vi "LVDimInterface.dic_info_service.vi"   [LabVIEW 2014, in "LVDimInterface.lvlib"]
uses:
  LVDimInterface.lvlib
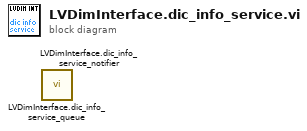
[diagram p0: block diagram]
diagram:
  n1 = call "LVDimInterface.dic_info_service_queue.vi"() -> ()  [unwired: 18 in, 2 out]
  n2 = call "LVDimInterface.dic_info_service_notifier.vi"() -> ()  [unwired: 18 in, 2 out]
